vi "Prime95BCameraSimpleOperationACQ.vi"(8 "error in (no error)":errorcluster, 11 "Config In":T1 {"Hardware Configuration"."Lasers Configuration"."SettingValues"."785 Power" format="%.1f"; "Hardware Configuration"."Lasers Configuration"."SettingValues"."647 Power" format="%.1f"; "Hardware Configuration"."Lasers Configuration"."SettingValues"."561 Power" format="%.1f"}) -> (0 "error out":errorcluster, 3 "Config Out":T1 {"Hardware Configuration"."Lasers Configuration"."SettingValues"."785 Power" format="%.1f"; "Hardware Configuration"."Lasers Configuration"."SettingValues"."647 Power" format="%.1f"; "Hardware Configuration"."Lasers Configuration"."SettingValues"."561 Power" format="%.1f"})   [LabVIEW 2019]
uses:
  C:/RM21-MMicrosopeSource/HardwareAdapter/Camera/Dependencies/PVCamNET.dll
  Dependencies/PVCamNET.dll
  Support/Hardware Configuration.ctl
  Logging/Logging Configuration.ctl
  Logging/Logging.lvlib
  Settings/System Running Settings.ctl
  Settings/Settings.lvlib
  Support/Camera Configuration.ctl
  controls/DeviceStatusCtl.ctl
  C:/RM21-MMicrosopeSource/HardwareAdapter/Lasers/Dependencies/Oxxius_Boxx.dll
  Lasers/Dependencies/Oxxius_Boxx.dll
  Controls/CallBack Refs.ctl
  <vilib>/vision/Image Controls.llb/IMAQ Image.ctl
panel:
  out "8 Bit Histogram":i32[](graph)
  in  "start":bool
  in  "stop":bool
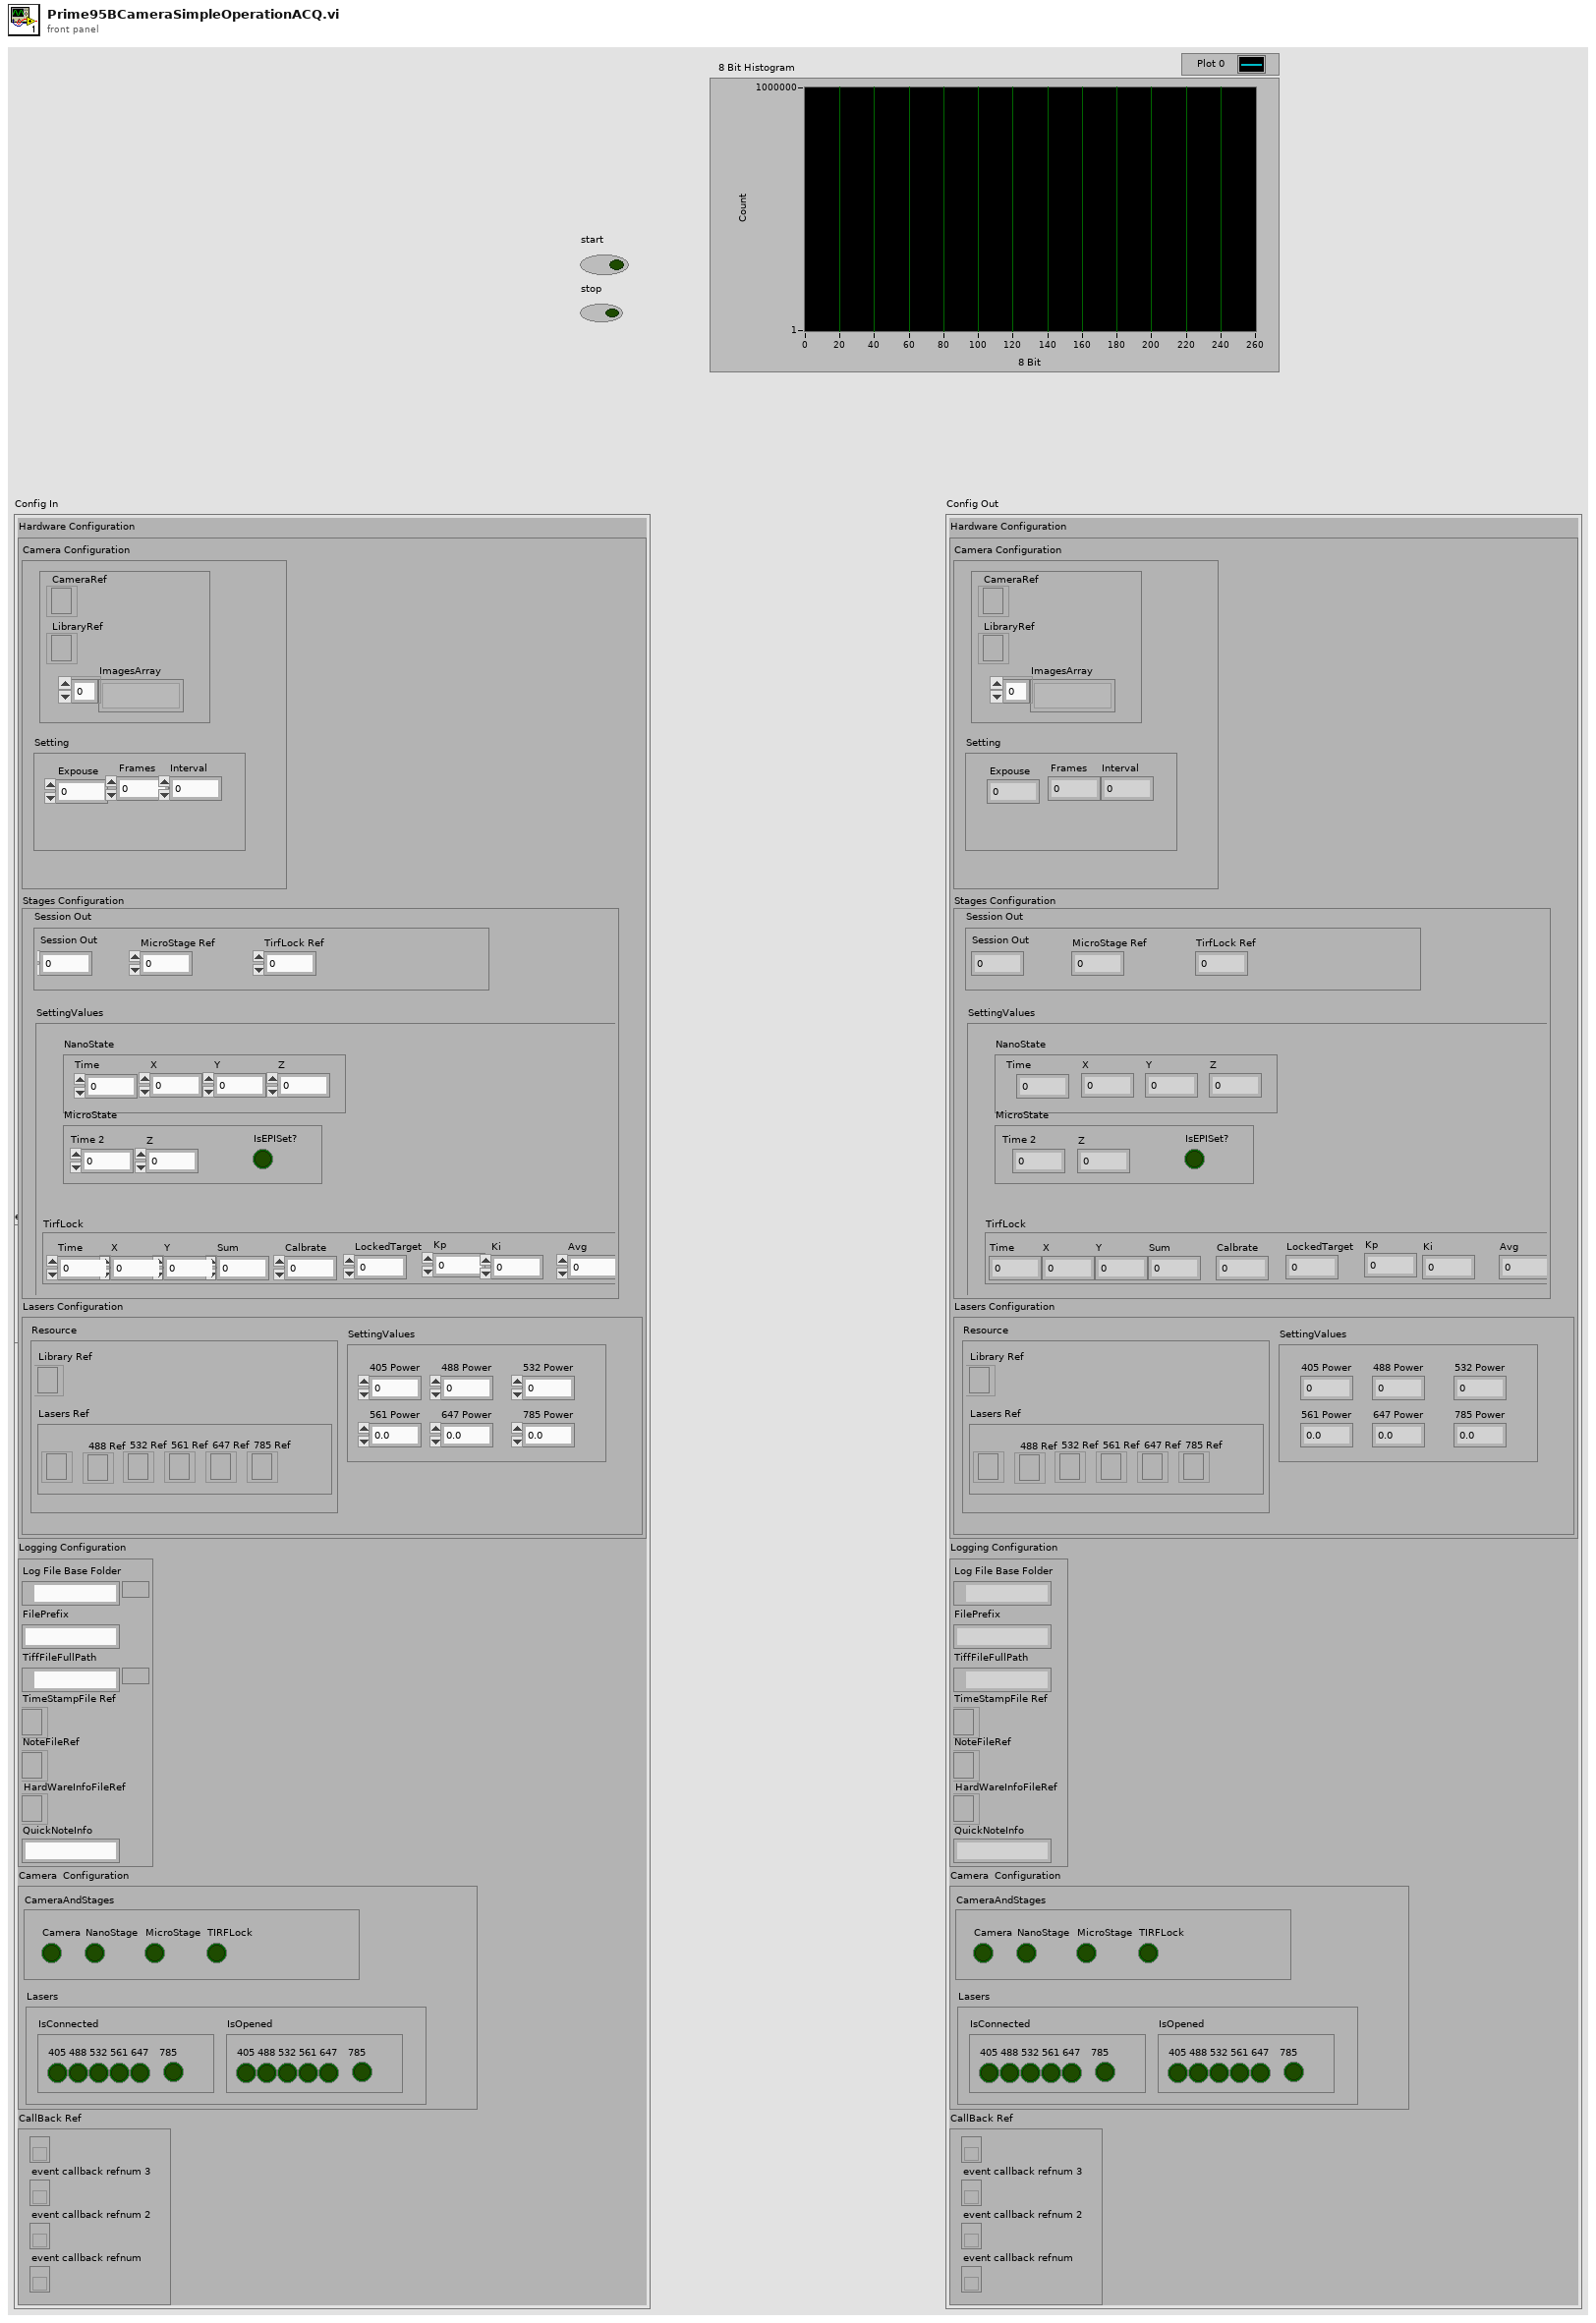
[diagram p1: front panel]
types:
  T1 = typedef "Settings.lvlib/System Running Settings.ctl" = cluster{"Hardware Configuration":T2, "Logging Configuration":T5, "HardWare Status":cluster{"CameraAndStages":T6, "Lasers":cluster{"IsConnected":cluster{"405":bool, "488":bool, "532":bool, "561":bool, "647":bool, "785":bool}, "IsOpened":cluster{"405":bool, "488":bool, "532":bool, "561":bool, "647":bool, "785":bool}}}, "CallBack Ref":T7}
  T2 = typedef "Hardware Configuration.ctl" = cluster{"Camera Configuration":T3, "Stages Configuration":cluster{"Resource":cluster{"NanoStage Ref":i32, "MicroStage Ref":i32, "TirfLock Ref":i32}, "SettingValues":cluster{"NanoState":cluster{"Time":dbl, "X":dbl, "Y":dbl, "Z":dbl}, "MicroState":cluster{"Time 2":dbl, "Z":dbl, "IsEPISet?":bool}, "TirfLock":cluster{"Time":dbl, "X":dbl, "Y":dbl, "Sum":dbl, "Calbrate":dbl, "LockedTarget":dbl, "Kp":dbl, "Ki":dbl, "Avg":dbl}}}, "Lasers Configuration":cluster{"SettingValues":cluster{"405 Power":sgl, "488 Power":sgl, "532 Power":sgl, "561 Power":sgl, "647 Power":sgl, "785 Power":sgl}, "Resource":cluster{"Library Ref":refnum<k24>, "Lasers Ref":cluster{"405 Ref":refnum<k24>, "488 Ref":refnum<k24>, "532 Ref":refnum<k24>, "561 Ref":refnum<k24>, "647 Ref":refnum<k24>, "785 Ref":refnum<k24>}}}}
  T3 = typedef "Camera Configuration.ctl" = cluster{"Setting":cluster{"Expouse":dbl, "Frames":dbl, "Interval":dbl}, "Resource":cluster{"CameraRef":refnum<k24>, "LibraryRef":refnum<k24>, "ImagesArray":T4[]}}
  T4 = typedef "IMAQ Image.ctl" = refnum<image>
  T5 = typedef "Logging.lvlib/Logging Configuration.ctl" = cluster{"Log File Base Folder":path, "FilePrefix":string, "TiffFileFullPath":path, "TimeStampFile Ref":refnum<file>, "NoteFileRef":refnum<file>, "HardWareInfoFileRef":refnum<file>, "QuickNoteInfo":string}
  T6 = typedef "DeviceStatusCtl.ctl" = cluster{"Camera":bool, "NanoStage":bool, "MicroStage":bool, "TIRFLock":bool}
  T7 = typedef "CallBack Refs.ctl" = cluster{"event callback refnum":refnum<k27>, "event callback refnum 2":refnum<k27>, "event callback refnum 3":refnum<k27>, "event callback refnum 4":refnum<k27>}
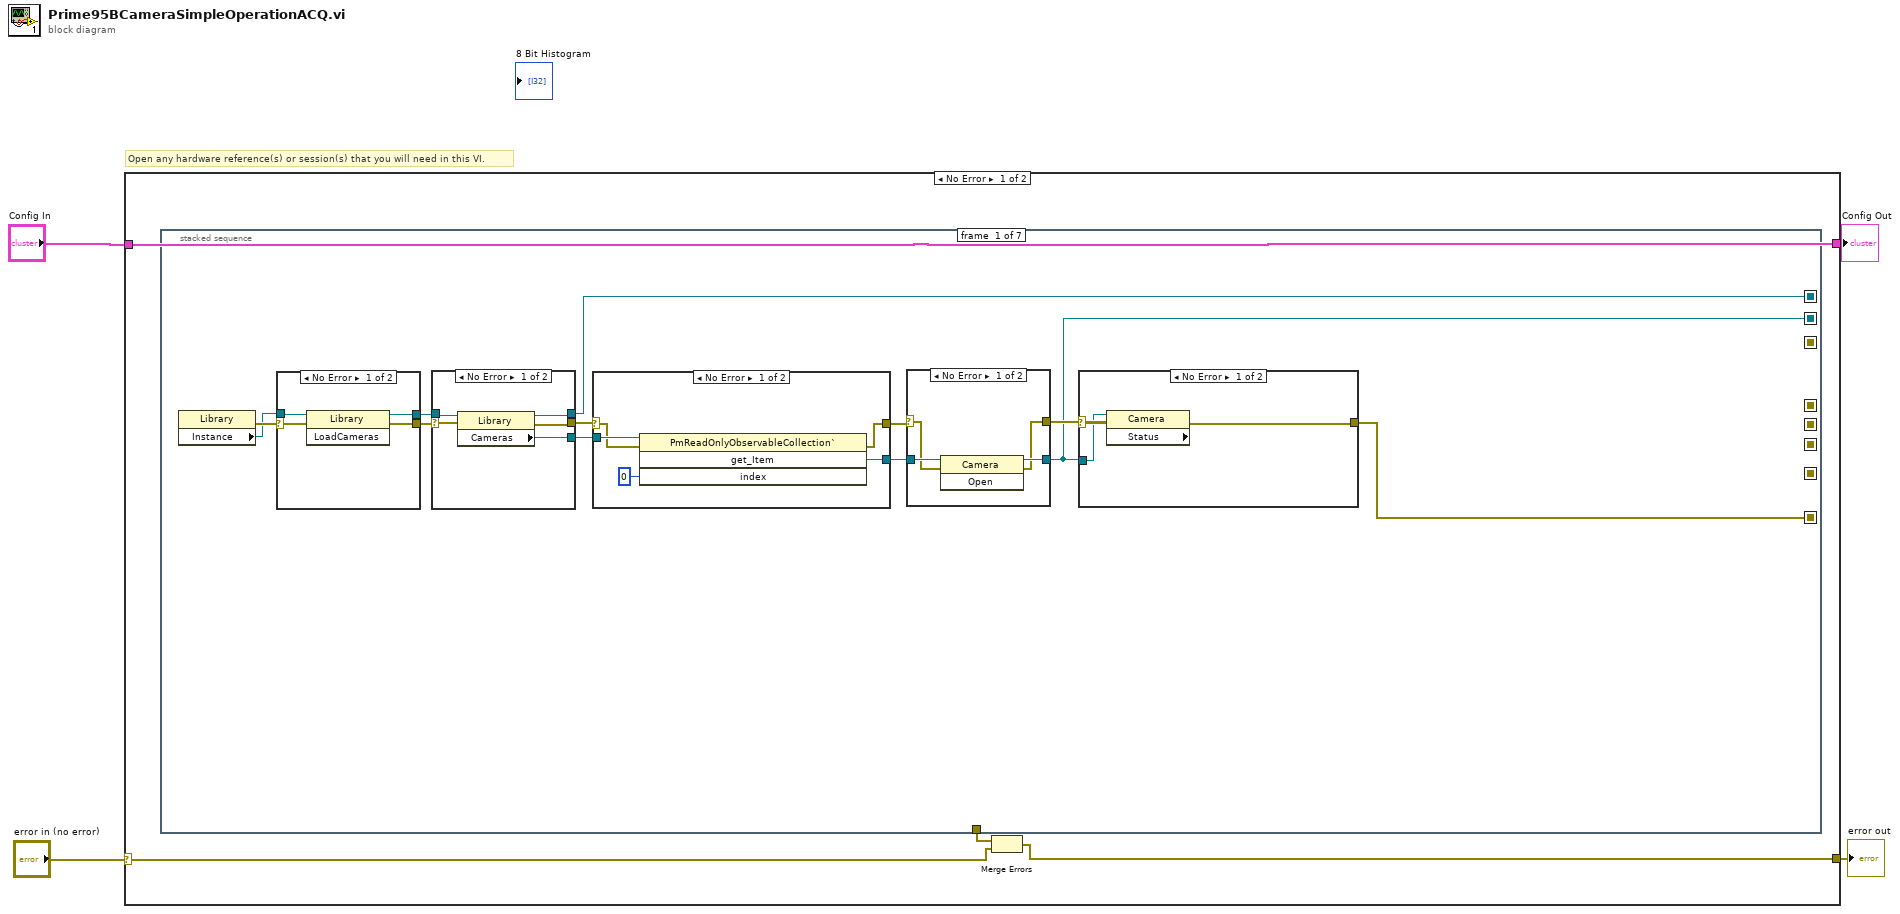
[diagram p0: block diagram]
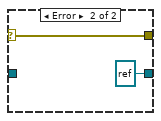
[diagram p3: hidden frame]
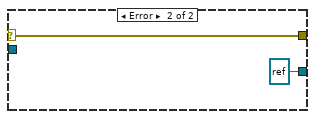
[diagram p4: hidden frame]
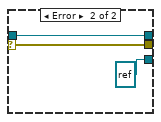
[diagram p5: hidden frame]
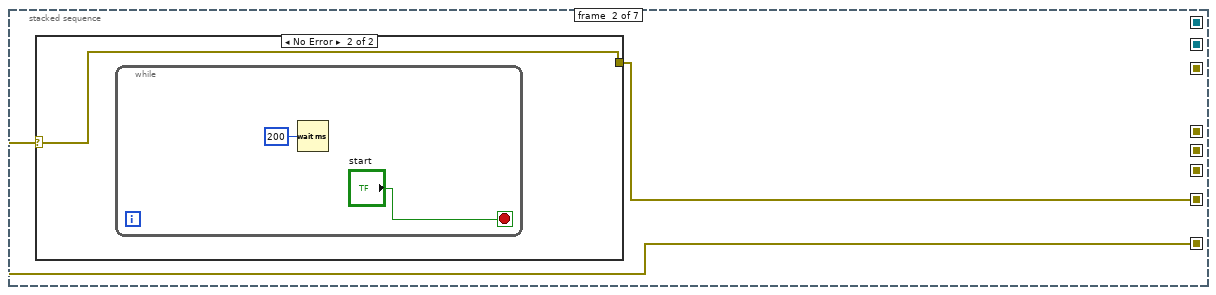
[diagram p7: hidden frame]
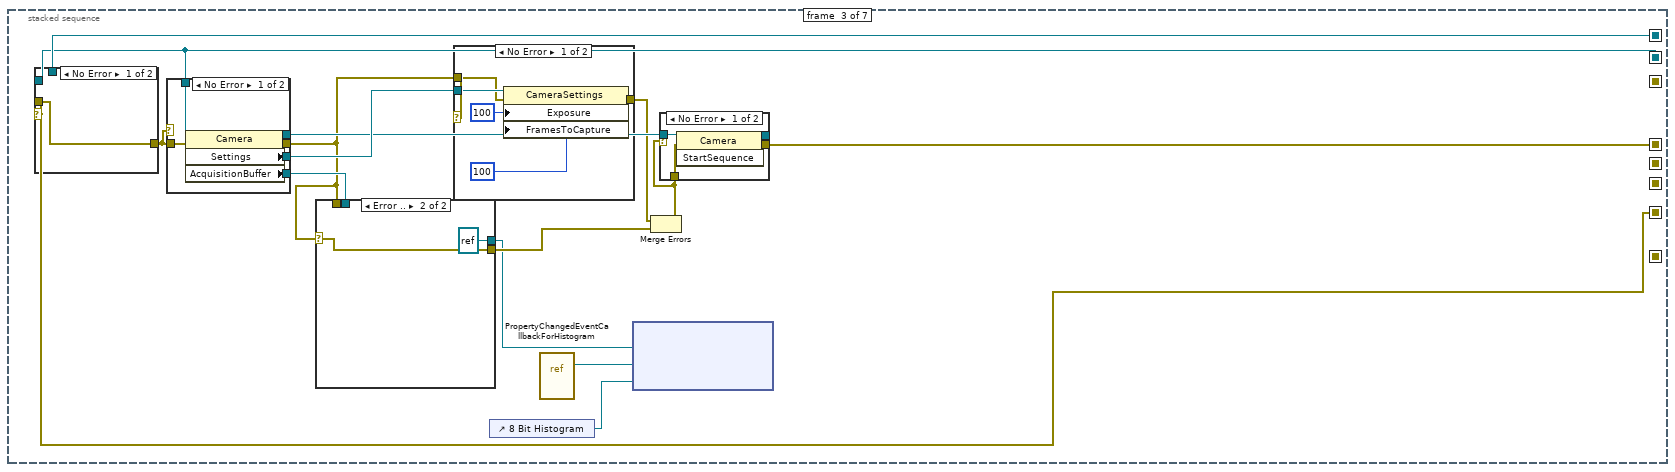
[diagram p9: hidden frame]
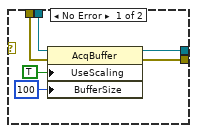
[diagram p12: hidden frame]
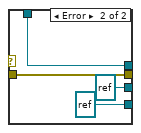
[diagram p13: hidden frame]
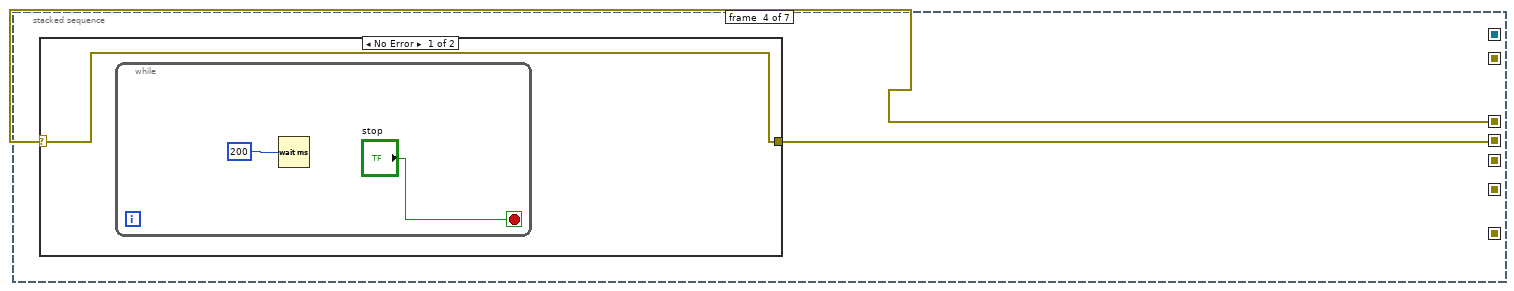
[diagram p15: hidden frame]
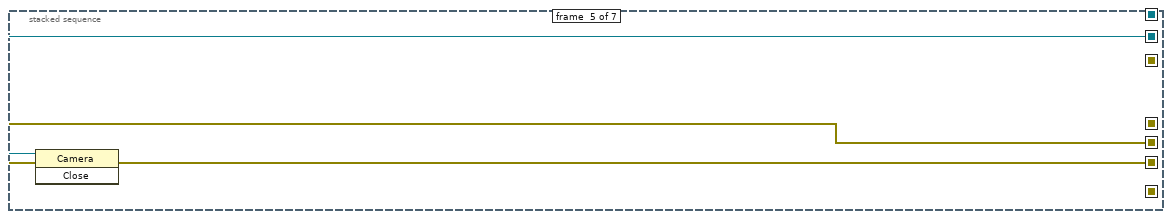
[diagram p17: hidden frame]
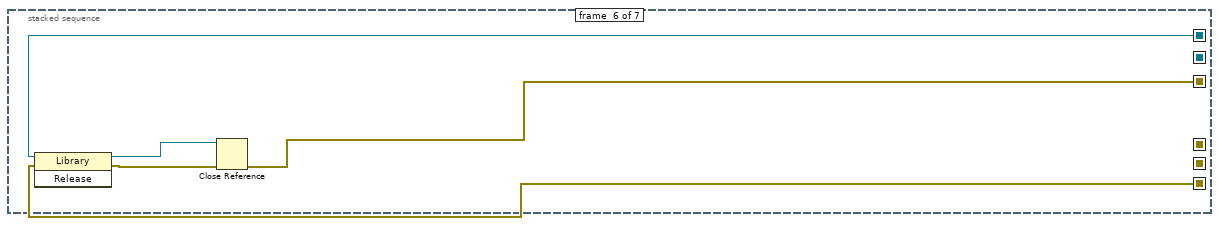
[diagram p18: hidden frame]
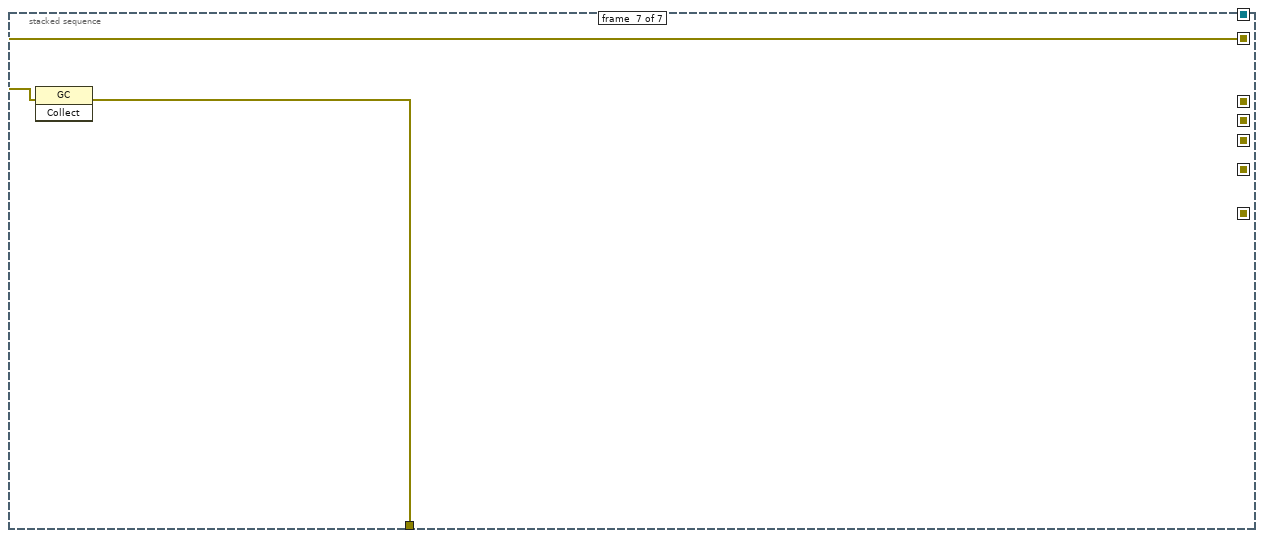
[diagram p19: hidden frame]
diagram:
  # "Open any hardware reference(s) or session(s) that you will need in this VI."
  n1 = case shown="No Error" "error in (no error)" {
    selector: "error in (no error)" -> [w6 w121]
    tunnel: [w5 w121] -> w3
    tunnel: "Config In" -> [w8 w122]
    tunnel: [w8 w122] -> w1
    frame No Error {
      n2 = stacked-sequence {
        seq-local: [w10 _ _ _ _ _ _] -> [_ w53 _ _ _ _ _]
        seq-local: [w9 _ _ _ _ _ _] -> [_ _ w69 _ w113 _ _]
        seq-local: [w12 _ _ _ _ _ _] -> [_ _ w72 _ _ w117 _]
        seq-local: [_ _ w61 _ _ _ _] -> [_ _ _ w106 _ _ _]
        seq-local: [_ _ _ _ w112 _ _] -> [_ _ _ _ _ w116 _]
        seq-local: [_ _ _ _ _ w114 _] -> [_ _ _ _ _ _ w120]
        seq-local: [_ w52 _ _ _ _ _] -> [_ _ w65 _ _ _ _]
        seq-local: [_ _ _ w105 _ _ _] -> [_ _ _ _ w111 _ _]
        tunnel: [_ _ _ _ _ _ w119] -> w7
        frame #0 {
          n3 = property class="Library"() -> (error out=w20:errorcluster, "Instance"=w17:refnum<k24>)  [unwired: 2 in, 1 out]
          n4 = case shown="No Error" w20 {
            selector: w20 -> [w47 w51]
            tunnel: [w48 w51] -> w18
            tunnel: [w49 w50] -> w19
            tunnel: w17 -> [w46 w50]
            frame No Error {
              n5 = invoke class="Library" method="LoadCameras"(reference=w46, error in=w47) -> (reference out=w49:refnum<k24>, error out=w48:errorcluster)  [unwired: 1 in, 1 out]
            }
            frame Error {
            }
          }
          n6 = case shown="No Error" w18 {
            selector: w18 -> [w42 w45]
            tunnel: [w39 w45] -> w14
            tunnel: w19 -> [w41 w44]
            tunnel: [w40 w44] -> w12
            tunnel: [w38 refnum<k24> refnum ("Cameras")] -> w16
            frame No Error {
              n7 = property class="Library"(reference=w41, error in=w42) -> (reference out=w40:refnum<k24>, error out=w39:errorcluster, "Cameras"=w38:refnum<k24>)
            }
            frame Error {
            }
          }
          n8 = case shown="No Error" w14 {
            selector: w14 -> [w32 w37]
            tunnel: w16 -> [w35 _]
            tunnel: [w33 refnum<k24> refnum ("get_Item")] -> w15
            tunnel: [w31 w37] -> w13
            frame No Error {
              n9 = invoke class="PmReadOnlyObservableCollection`" method="get_Item"(reference=w35, error in=w32, "index"=0) -> (error out=w31:errorcluster, "get_Item"=w33:refnum<k24>)  [unwired: 1 in, 2 out]
            }
            frame Error {
            }
          }
          n10 = case shown="No Error" w13 {
            selector: w13 -> [w26 w30]
            tunnel: [w25 w30] -> w11
            tunnel: w15 -> [w28 _]
            tunnel: [w27 refnum<k24> refnum ("get_Item")] -> w9
            frame No Error {
              n11 = invoke class="Camera" method="Open"(reference=w28, error in=w26) -> (reference out=w27:refnum<k24>, error out=w25:errorcluster)  [unwired: 1 in, 1 out]
            }
            frame Error {
            }
          }
          n12 = case shown="No Error" w11 {
            selector: w11 -> [w22 w24]
            tunnel: [w21 w24] -> w10
            tunnel: w9 -> [w23 _]
            frame No Error {
              n13 = property class="Camera" props=["Status"](reference=w23, error in=w22) -> (error out=w21:errorcluster)  [unwired: 2 out]
            }
            frame Error {
            }
          }
        }
        frame #1 {
          n14 = case shown="No Error" w53 {
            selector: w53 -> [w54 w55]
            tunnel: [w54 w55] -> w52
            frame Error {
            }
            frame No Error {
              n15 = while {
                stop <- "start" stop-if-true
                n16 = Wait (ms)(milliseconds to wait=u32 200) -> ()  [unwired: 1 out]
              }
            }
          }
        }
        frame #2 {
          n17 = case shown="No Error" w65 {
            tunnel: w72 -> [_ _]
            tunnel: [w103 w104] -> w64
            tunnel: w69 -> [_ _]
            tunnel: w65 -> [w103 w104]
            frame No Error {
            }
            frame Error {
            }
          }
          n18 = case shown="No Error" w64 {
            tunnel: [w98 refnum<k24> refnum ("Settings")] -> w71
            tunnel: [w97 refnum<k24> refnum ("AcquisitionBuffer")] -> w70
            tunnel: w64 -> [w96 w102]
            tunnel: w69 -> [w95 w101]
            tunnel: [w94 w101] -> w68
            tunnel: [w93 w102] -> w63
            frame No Error {
              n19 = property class="Camera"(reference=w95, error in=w96) -> (reference out=w94:refnum<k24>, error out=w93:errorcluster, "Settings"=w98:refnum<k24>, "AcquisitionBuffer"=w97:refnum<k24>)
            }
            frame Error {
            }
          }
          n20 = case shown="Error .." w63 {
            selector: w63 -> [_ w92]
            tunnel: w70 -> [w90 _]
            tunnel: w63 -> [w88 _]
            tunnel: [w87 w92] -> w66
            tunnel: [w85 refnum<k24> refnum ("AcquisitionBuffer")] -> w60
            frame No Error {
              n21 = property class="AcqBuffer"(reference=w90, error in=w88, "UseScaling"=TRUE, "BufferSize"=100) -> (reference out=w85:refnum<k24>, error out=w87:errorcluster)
            }
            frame Error {
            }
          }
          n22 = case shown="No Error" w63 {
            tunnel: w71 -> [w83 _]
            tunnel: [w82 w84] -> w67
            tunnel: w63 -> [w81 w84]
            frame No Error {
              n23 = property class="CameraSettings"(reference=w83, error in=w81, "Exposure"=u32 100, "FramesToCapture"=u16 100) -> (error out=w82:errorcluster)  [unwired: 1 out]
            }
            frame Error {
            }
          }
          n24 = control-ref of="8 Bit Histogram"() -> (w58:refnum<vi>)
          n25 = vi-ref "PropertyChangedEventCallbackForHistogram.vi"() -> ("vi reference"=w59:refnum<vi>)
          n26 = node(w60, w59, w58) -> ()  [unwired: 2 in, 2 out]
          n27 = Merge Errors(w67, w66) -> (w62:errorcluster)
          n28 = case shown="No Error" w62 {
            selector: w62 -> [_ w78]
            tunnel: w68 -> [w76 w77]
            tunnel: [w75 w78] -> w61
            tunnel: [w74 w77] -> _
            tunnel: w62 -> [w73 _]
            frame No Error {
              n29 = invoke class="Camera" method="StartSequence"(reference=w76, error in=w73) -> (reference out=w74:refnum<k24>, error out=w75:errorcluster)  [unwired: 1 in, 1 out]
            }
            frame Error {
            }
          }
        }
        frame #3 {
          n30 = case shown="No Error" w106 {
            selector: w106 -> [w107 w110]
            tunnel: [w107 w110] -> w105
            frame No Error {
              n31 = while {
                stop <- "stop" stop-if-true
                n32 = Wait (ms)(milliseconds to wait=u32 200) -> ()  [unwired: 1 out]
              }
            }
            frame Error {
            }
          }
        }
        frame #4 {
          n33 = invoke class="Camera" method="Close"(reference=w113, error in=w111) -> (error out=w112:errorcluster)  [unwired: 1 in, 2 out]
        }
        frame #5 {
          n34 = invoke class="Library" method="Release"(reference=w117, error in=w116) -> (reference out=w118:refnum<k24>, error out=w115:errorcluster)  [unwired: 1 in, 1 out]
          n35 = Close Reference(reference=w118, error in (no error)=w115) -> (error out=w114:errorcluster)
        }
        frame #6 {
          n36 = invoke class="GC" method="Collect"(error in=w120) -> (error out=w119:errorcluster)  [unwired: 2 in, 2 out]
        }
      }
      n37 = Merge Errors(w7, w6) -> (w5:errorcluster)
    }
    frame Error {
    }
  }
  "error out" <- w3
  "Config Out" <- w1
